vi "BinRemoval.vi"(8 "error in (no error)":errorcluster, 11 "Node Ptr":u64 format="%.0x") -> (0 "error out":errorcluster)   [LabVIEW 2012, in "Histogram Custom Device.lvlib"]
uses:
  Histogram Custom Device.lvlib
  <vilib>/NI Veristand/Custom Device API/Custom Device API.lvlib
  <vilib>/NI Veristand/Custom Device API/Get Item Property (Variant).vi
  BinBounds.ctl
  <vilib>/NI Veristand/Custom Device API/Custom Device Channel Type.ctl
  <vilib>/NI Veristand/Custom Device API/Set Item Property (Variant).vi
panel:
  in  "Tag":string
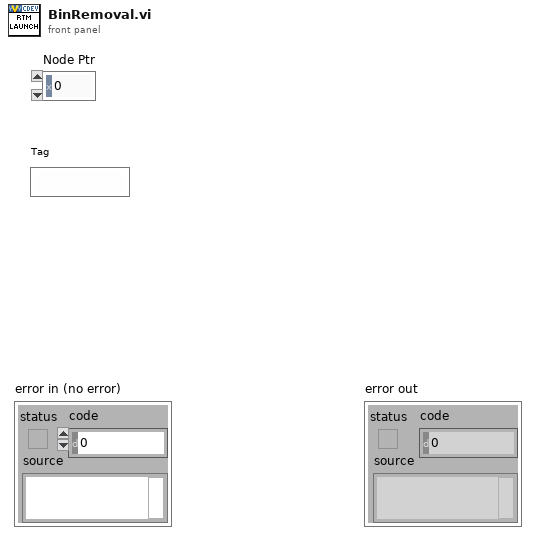
[diagram p1: front panel]
types:
  T1 = typedef "Custom Device API.lvlib/Custom Device Channel Type.ctl" = enum16{"Input", "Output"}
  T2 = typedef "Histogram Custom Device.lvlib/BinBounds.ctl" = cluster{"Bin Counts":i32[], "Upper Bounds":dbl[], "Lower Bounds":dbl[]}
  T3 = typedef "Custom Device API.lvlib/Custom Device Item Ref.ctl" = u64
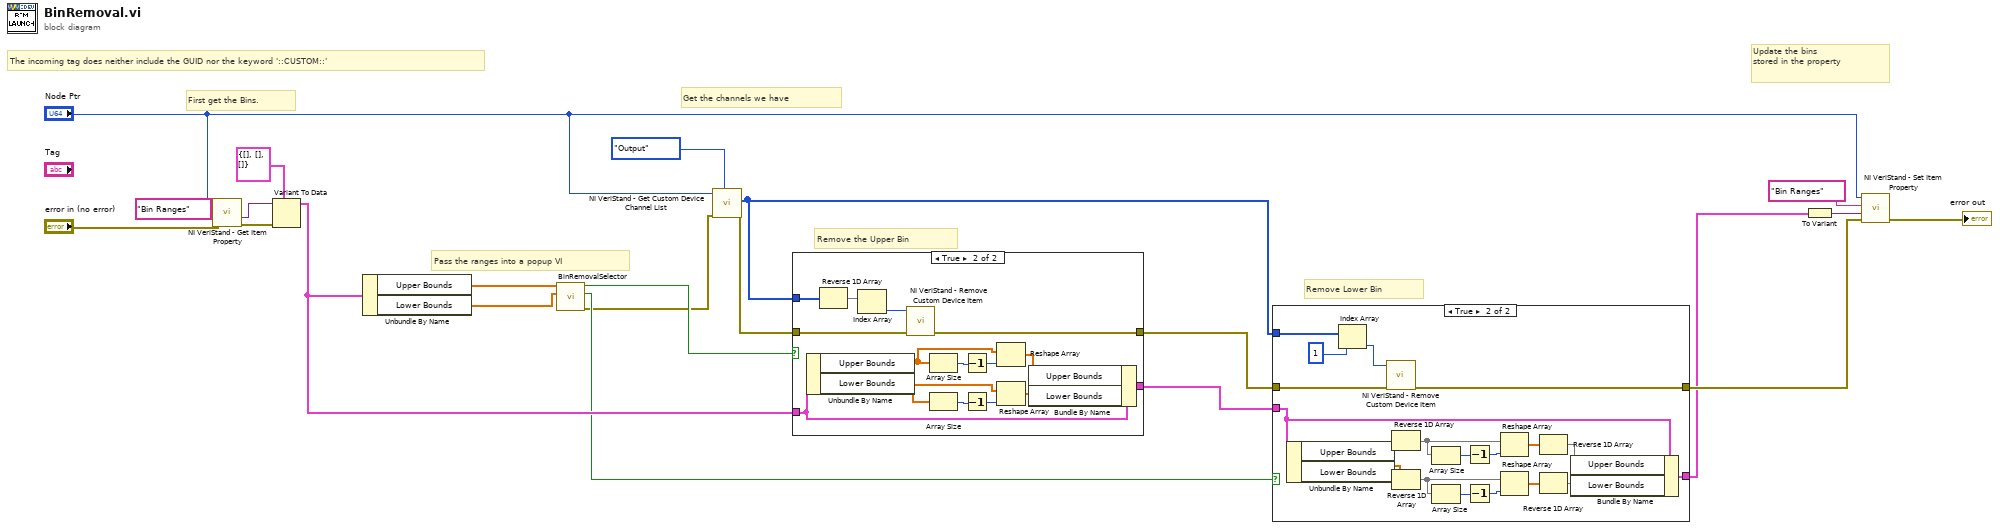
[diagram p0: block diagram]
diagram:
  # "Update the bins\nstored in the property"
  # "Remove the Upper Bin"
  # "Get the channels we have"
  # "Remove Lower Bin"
  # "Pass the ranges into a popup VI"
  # "First get the Bins."
  # "The incoming tag does neither include the GUID nor the keyword '::CUSTOM::'"
  n1 = call-poly <vilib>:"NI VeriStand - Get Item Property.vi"("error in (no error)"="error in (no error)", "Property Name"="Bin Ranges", "Item Ref in"="Node Ptr") -> ("error out"=w21:errorcluster, "Value"=w22:variant)  [unwired: 5 in, 2 out]
  n2 = Variant To Data(error in=w21, type=T2 {"Bin Counts"=[], "Upper Bounds"=[], "Lower Bounds"=[]} ("Cluster"), Variant=w22) -> (data=w11:T2)  [unwired: 1 out]
  n3 = Unbundle By Name(w11) -> ("Upper Bounds"=w5:dbl[], "Lower Bounds"=w4:dbl[])
  n4 = call "BinRemovalSelector.vi"("Lower Bounds"=w4, "Upper Bounds"=w5) -> ("error out"=w1:errorcluster, "RemoveLowestBin"=w2:bool, "RemoveHighestBin"=w3:bool)  [unwired: 7 in]
  n5 = call <vilib>:"NI VeriStand - Get Custom Device Channel List.vi"("Channel Type"=Custom_Device_Channel_Type."Output", "error in (no error)"=w1, "Device Ref in"="Node Ptr") -> ("error out"=w16:errorcluster, "Specified Channel Ref List"=w15:T3[])  [unwired: 6 in, 1 out]
  n6 = case shown="True" w3 {
    tunnel: w15 -> [_ w39]
    tunnel: w16 -> [w24 w36]
    tunnel: [w24 w35] -> w14
    tunnel: w11 -> [w23 w31]
    tunnel: [w23 w25] -> w7
    frame False {
    }
    frame True {
      n7 = Unbundle By Name(w31) -> ("Upper Bounds"=w32:dbl[], "Lower Bounds"=w27:dbl[])
      n8 = Reverse 1D Array(array=w39) -> (reversed array=w38:T3[])
      n9 = Index Array(array=w38) -> (element=w37:T3)  [unwired: 1 in]
      n10 = call <vilib>:"NI VeriStand - Remove Custom Device Item.vi"("error in (no error)"=w36, "Item Ref in"=w37) -> ("error out"=w35:errorcluster)  [unwired: 8 in, 1 out]
      n11 = Array Size(array=w32) -> (size(s)=w34:i32)
      n12 = Array Size(array=w27) -> (size(s)=w28:i32)
      n13 = Decrement(x=w34) -> (x-1=w33:i32)
      n14 = Decrement(x=w28) -> (x-1=w29:i32)
      n15 = Reshape Array(w32, w33) -> (w30:dbl[])
      n16 = Reshape Array(w27, w29) -> (w26:dbl[])
      n17 = Bundle By Name(cluster=w31, "Upper Bounds"=w30, "Lower Bounds"=w26) -> (w25:T2)
    }
  }
  n18 = case shown="True" w2 {
    tunnel: w15 -> [_ w58]
    tunnel: [w41 w59] -> w13
    tunnel: w14 -> [w41 w56]
    tunnel: w7 -> [w40 w42]
    tunnel: [w40 w43] -> w6
    frame False {
    }
    frame True {
      n19 = Unbundle By Name(w42) -> ("Upper Bounds"=w50:dbl[], "Lower Bounds"=w54:dbl[])
      n20 = Index Array(array=w58, index=1) -> (element=w60:T3)
      n21 = call <vilib>:"NI VeriStand - Remove Custom Device Item.vi"("error in (no error)"=w56, "Item Ref in"=w60) -> ("error out"=w59:errorcluster)  [unwired: 8 in, 1 out]
      n22 = Reverse 1D Array(array=w50) -> (reversed array=w46:dbl[])
      n23 = Reverse 1D Array(array=w54) -> (reversed array=w47:dbl[])
      n24 = Array Size(array=w46) -> (size(s)=w48:i32)
      n25 = Array Size(array=w47) -> (size(s)=w53:i32)
      n26 = Decrement(x=w48) -> (x-1=w49:i32)
      n27 = Decrement(x=w53) -> (x-1=w52:i32)
      n28 = Reshape Array(w46, w49) -> (w51:dbl[])
      n29 = Reshape Array(w47, w52) -> (w55:dbl[])
      n30 = Reverse 1D Array(array=w51) -> (reversed array=w45:dbl[])
      n31 = Reverse 1D Array(array=w55) -> (reversed array=w44:dbl[])
      n32 = Bundle By Name(cluster=w42, "Upper Bounds"=w45, "Lower Bounds"=w44) -> (w43:T2)
    }
  }
  n33 = To Variant(anything=w6) -> (Variant=w10:variant)
  n34 = call-poly <vilib>:"NI VeriStand - Set Item Property.vi"("error in (no error)"=w13, "Value"=w10, "Property Name"="Bin Ranges", "Item Ref in"="Node Ptr") -> ("error out"=→"error out":errorcluster)  [unwired: 5 in, 2 out]
